vi "XY Graph Get Tail (& Head) & Extra Points for Extrapolated Decay.vi"(0 "# Additional Points":i32, 1 "Tail Fraction":dbl, 2 "Head Fraction":dbl, 5 "X Array":dbl[](array[numeric]), 7 "Y Array":dbl[](array[numeric]), 9 "Overweight Head":bool, 11 "Error In":errorcluster, 12 "Periodic Decay":bool, 13 "Period":dbl=0.5) -> (4 "Additional Tail Points":dbl[](array[numeric]), 6 "X Array to Fit":dbl[](array[numeric]), 8 "Y Array to Fit":dbl[](array[numeric]), 10 "Weight Array":dbl[](array[numeric]), 15 "Error Out":errorcluster)   [LabVIEW 2021, in "XY Graph Add-Ons.lvlib"]
uses:
  XY Graph Add-Ons.lvlib
  <vilib>/gmath/statdist.llb/st_Percentiles (scalar).vi
  <vilib>/Utility/error.llb/Error Cluster From Error Code.vi
  <vilib>/ErrorRing/Error Ring.xnode
  Arrays/Arrays.lvlib
  <vilib>/gmath/NI_Gmath.lvlib
  8a88247f-15af-4228-96b1-d00a8001144d.vi
panel:
  out "percentile":dbl
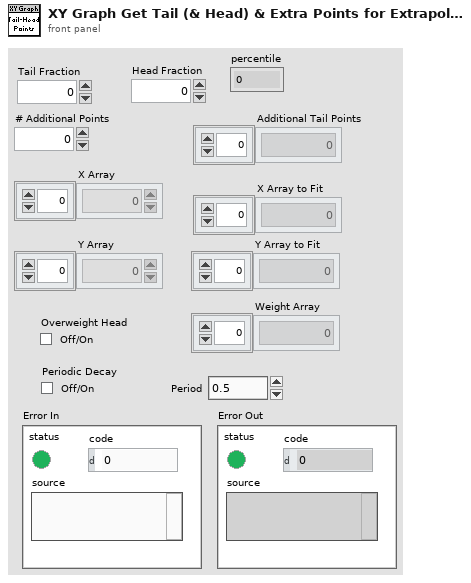
[diagram p1: front panel]
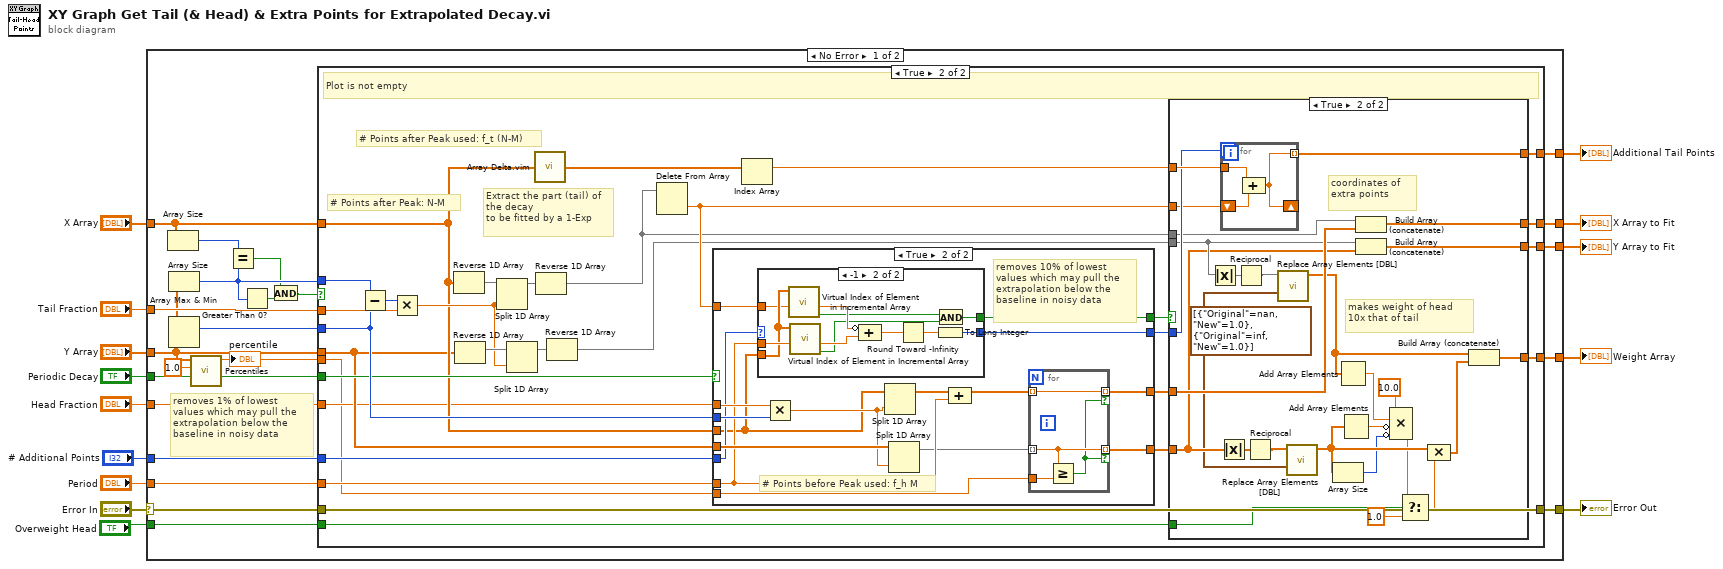
[diagram p0: block diagram]
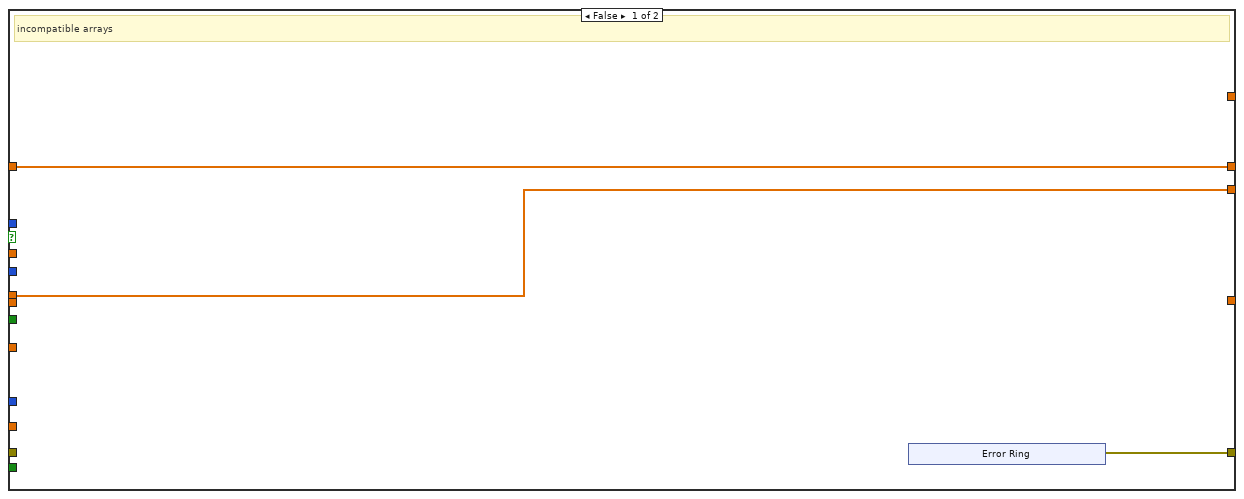
[diagram p2: hidden frame]
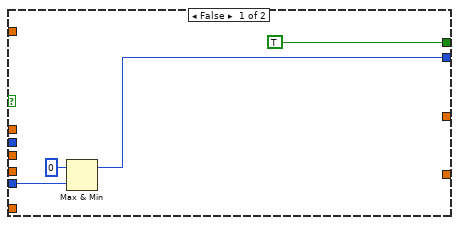
[diagram p4: hidden frame]
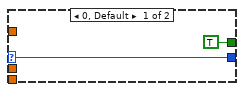
[diagram p5: hidden frame]
diagram:
  n1 = case shown="No Error" "Error In" {
    selector: "Error In" -> [w24 w144]
    tunnel: "Y Array" -> [w17 w142]
    tunnel: [w36 w143] -> w5
    tunnel: "# Additional Points" -> [w35 _]
    tunnel: [w34 _] -> w12
    tunnel: "Tail Fraction" -> [w32 _]
    tunnel: [w31 w142] -> w4
    tunnel: "X Array" -> [w30 w143]
    tunnel: [w23 w144] -> w8
    tunnel: "Periodic Decay" -> [w22 _]
    tunnel: "Period" -> [w21 _]
    tunnel: "Head Fraction" -> [w20 _]
    tunnel: [w19 _] -> w2
    tunnel: "Overweight Head" -> [w18 _]
    frame No Error {
      # "removes 1% of lowest values which may pull the extrapolation below the baseline in noisy data"
      n2 = Array Size(array=w30) -> (size(s)=w29:i32)
      n3 = Array Size(array=w17) -> (size(s)=w28:i32)
      n4 = Array Max & Min(array=w17) -> (max index (indices)=w33:i32)  [unwired: 3 out]
      n5 = call-poly <vilib>:"Percentiles.vi"("p"=1.0, "x array"=w17) -> ("percentile"=w15:dbl)  [unwired: 8 in, 1 out]
      "percentile" <- w15
      n6 = Equal?(x=w29, y=w28) -> (x = y?=w26:bool)
      n7 = Greater Than 0?(x=w28) -> (x > 0?=w27:bool)
      n8 = And(x=w26, y=w27) -> (x .and. y?=w25:bool)
      n9 = case shown="True" w25 {
        tunnel: w17 -> [w38 w56]
        tunnel: [w39 w59] -> w36
        tunnel: w35 -> [_ w52]
        tunnel: [_ w60] -> w34
        tunnel: w33 -> [_ w63]
        tunnel: w32 -> [_ w64]
        tunnel: [w38 w58] -> w31
        tunnel: w30 -> [w39 w57]
        tunnel: w28 -> [_ w66]
        tunnel: w24 -> [_ w65]
        tunnel: [w37 w65] -> w23
        tunnel: w22 -> [_ w62]
        tunnel: w21 -> [_ w61]
        tunnel: w20 -> [_ w53]
        tunnel: [_ w46] -> w19
        tunnel: w18 -> [_ w45]
        tunnel: w15 -> [_ w44]
        frame False {
          # "incompatible arrays"
          n10 = xnode "Error Ring"() -> ("error out"=w37:errorcluster)
        }
        frame True {
          # "# Points after Peak: N-M"
          # "Extract the part (tail) of the decay\nto be fitted by a 1-Exp"
          # "Plot is not empty"
          # "# Points after Peak used: f_t (N-M)"
          n11 = Subtract(x=w66, y=w63) -> (x-y=w72:i32)
          n12 = Multiply(x=w72, y=w64) -> (x*y=w68:dbl)
          n13 = Reverse 1D Array(array=w57) -> (reversed array=w71:dbl[])
          n14 = Reverse 1D Array(array=w56) -> (reversed array=w69:dbl[])
          n15 = Split 1D Array(array=w71, index=w68) -> (first subarray=w70:dbl[])  [unwired: 1 out]
          n16 = Split 1D Array(array=w69, index=w68) -> (first subarray=w67:dbl[])  [unwired: 1 out]
          n17 = call "Array Delta.vim"("A[i]"=w57) -> ("A[i+1]-A[i]"=w73:dbl[])  [unwired: 8 in]
          n18 = Reverse 1D Array(array=w70) -> (reversed array=w49:dbl[])
          n19 = Reverse 1D Array(array=w67) -> (reversed array=w48:dbl[])
          n20 = Delete From Array(array=w49) -> (deleted portion=w50:dbl)  [unwired: 2 in, 1 out]
          n21 = case shown="True" w62 {
            tunnel: w53 -> [_ w124]
            tunnel: w63 -> [_ w123]
            tunnel: w61 -> [_ w117]
            tunnel: w57 -> [_ w116]
            tunnel: w56 -> [_ w122]
            tunnel: [_ w109] -> w55
            tunnel: [_ w110] -> w54
            tunnel: w52 -> [w108 w119]
            tunnel: [w106 w118] -> w51
            tunnel: w50 -> [_ w115]
            tunnel: [TRUE w114] -> w47
            tunnel: w44 -> [_ w111]
            frame False {
              n22 = Max & Min(x=0, y=w108) -> (max(x,y)=w106:i32)  [unwired: 1 out]
            }
            frame True {
              # "removes 10% of lowest values which may pull the extrapolation below the baseline in noisy data"
              # "# Points before Peak used: f_h M"
              n23 = case shown="-1" w119 {
                selector: w119 -> [w130 _]
                tunnel: [w130 w134] -> w118
                tunnel: w117 -> [_ w141]
                tunnel: w116 -> [_ w140]
                tunnel: w115 -> [_ w139]
                tunnel: [TRUE w131] -> w114
                frame 0, Default {
                }
                frame -1 {
                  n24 = call "Virtual Index of Element in Incremental Array.vi"("Value"=w139, "Incremental Array"=w140) -> ("Valid Array"=w133:bool, "Virtual Index"=w138:dbl)  [unwired: 8 in]
                  n25 = call "Virtual Index of Element in Incremental Array.vi"("Value"=w141, "Incremental Array"=w140) -> ("Valid Array"=w132:bool, "Virtual Index"=w137:dbl)  [unwired: 8 in]
                  n26 = Compound Arithmetic op=ADD(invert w138, w137) -> (w136:dbl)
                  n27 = Round Toward -Infinity(1:w136) -> (0:w135:dbl)
                  n28 = To Long Integer(number=w135) -> (32bit integer=w134:i32)
                  n29 = And(x=w133, y=w132) -> (x .and. y?=w131:bool)
                }
              }
              n30 = Multiply(x=w124, y=w123) -> (x*y=w121:dbl)
              n31 = Split 1D Array(array=w116, index=w121) -> (first subarray=w120:dbl[])  [unwired: 1 out]
              n32 = Split 1D Array(array=w122, index=w121) -> (first subarray=w113:dbl[])  [unwired: 1 out]
              n33 = Compound Arithmetic op=ADD(w120, w117) -> (w112:dbl[])
              n34 = for {
                tunnel: w113 -> [w127] mode=indexing
                tunnel: w112 -> [w126] mode=indexing
                tunnel: w111 -> [w128]
                tunnel: [w127] -> w110 mode=indexing if=w125
                tunnel: [w126] -> w109 mode=indexing if=w125
                n35 = Greater Or Equal?(x=w127, y=w128) -> (x >= y?=w125:bool)
              }
            }
          }
          n36 = Index Array(array=w73) -> (element=w74:dbl)  [unwired: 1 in]
          n37 = case shown="True" w47 {
            tunnel: w74 -> [_ w101]
            tunnel: [_ w100] -> w60
            tunnel: [_ w84] -> w59
            tunnel: [_ w83] -> w58
            tunnel: w55 -> [_ w99]
            tunnel: w54 -> [_ w90]
            tunnel: w51 -> [_ w98]
            tunnel: w50 -> [_ w97]
            tunnel: w49 -> [_ w96]
            tunnel: w48 -> [_ w93]
            tunnel: [_ w82] -> w46
            tunnel: w45 -> [_ w86]
            frame False {
              # "invalid array"
            }
            frame True {
              w89 = cluster{"Original":dbl, "New":dbl}[] [{"Original"=nan, "New"=1.0}, {"Original"=inf, "New"=1.0}] ("Array of Replacement Pairs")
              # "makes weight of head 10x that of tail"
              # "coordinates of extra points"
              n38 = Absolute Value(x=w93) -> (abs(x)=w95:dbl[])
              n39 = Absolute Value(x=w90) -> (abs(x)=w91:dbl[])
              n40 = for {
                N: w98 -> [_]
                shift-right: [w102] -> _
                shift-left: w97 -> [w103]
                tunnel: w101 -> [w104]
                tunnel: [w102] -> w100 mode=indexing
                n41 = Compound Arithmetic op=ADD(w104, w103) -> (w102:dbl)
              }
              n42 = Reciprocal(x=w95) -> (1/x=w94:dbl[])
              n43 = Reciprocal(x=w91) -> (1/x=w92:dbl[])
              n44 = call "Replace Array Elements [DBL].vi"("Array of Replacement Pairs"=w89, "Array"=w94) -> ("Array with Replacements"=w81:dbl[])  [unwired: 8 in, 1 out]
              n45 = call "Replace Array Elements [DBL].vi"("Array of Replacement Pairs"=w89, "Array"=w92) -> ("Array with Replacements"=w78:dbl[])  [unwired: 8 in, 1 out]
              n46 = Array Size(array=w78) -> (size(s)=w77:i32)
              n47 = Add Array Elements(numeric array=w81) -> (sum=w79:dbl)
              n48 = Add Array Elements(numeric array=w78) -> (sum=w80:dbl)
              n49 = Build Array (concatenate)(w96, w99) -> (w84:dbl[])
              n50 = Build Array (concatenate)(w93, w90) -> (w83:dbl[])
              n51 = Compound Arithmetic op=MULTIPLY(10.0 ("value"), w79, invert w80, invert w77) -> (w76:dbl)
              n52 = Select(t=w76, s=w86, f=1.0) -> (s? t:f=w87:dbl)
              n53 = Compound Arithmetic op=MULTIPLY(w78, w87) -> (w88:dbl[])
              n54 = Build Array (concatenate)(w81, w88) -> (w82:dbl[])
            }
          }
        }
      }
    }
    frame Error {
    }
  }
  "Y Array to Fit" <- w4
  "Additional Tail Points" <- w12
  "X Array to Fit" <- w5
  "Error Out" <- w8
  "Weight Array" <- w2
